vi "CallDLL.vi"() -> ()   [LabVIEW 2013]
uses:
  builds/SenslessProject/Meine DLL/SharedLib.dll
  Windows/System32/kernel32.dll
panel:
  out "String":string
  out "Fehler (Ausgang) 2":errorcluster caption="Fehler (Ausgang)"
  out "arg2":u32
  out "arg1":u32
  out "Fehler (Ausgang)":errorcluster
  out "Rückgabetyp":i32
  out "string_ 2":string
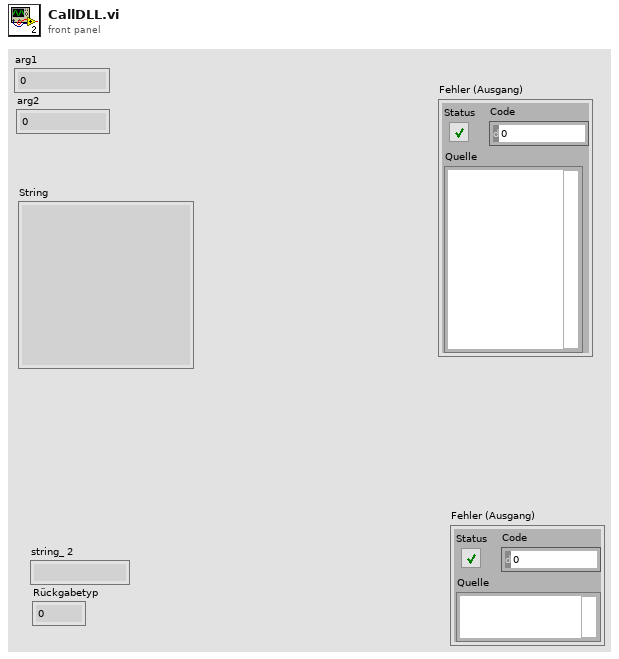
[diagram p1: front panel]
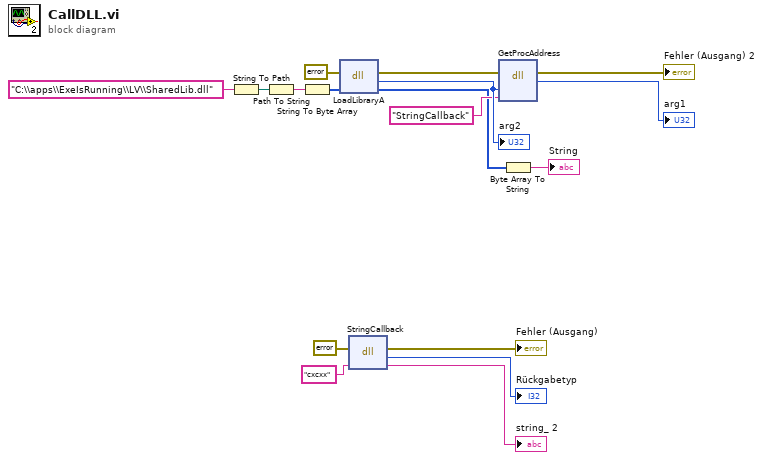
[diagram p0: block diagram]
diagram:
  n1 = String To Path(string="C:\\apps\\ExeIsRunning\\LV\\SharedLib.dll" ("arg1")) -> (path=w14:path)
  n2 = Path To String(path=w14) -> (string=w16:string)
  n3 = String To Byte Array(string=w16) -> (unsigned byte array=w17:u8[])
  n4 = dll-call lib="C:/Windows/System32/kernel32.dll" fn="LoadLibraryA"(error in=errorcluster {"status"=FALSE, "code"=0, "source"=""} ("Fehler (Eingang, kein Fehler)"), "arg1"=w17) -> (error out=w10:errorcluster, "Rückgabetyp"=w13:u32, "arg1"=w3:u8[])  [unwired: 2 in, 1 out]
  "arg2" <- w13
  n5 = dll-call lib="C:/apps/ExeIsRunning/builds/SenslessProject/Meine DLL/SharedLib.dll" fn="StringCallback"(error in=errorcluster {"status"=FALSE, "code"=0, "source"=""} ("Fehler (Eingang, kein Fehler)"), "string_"="cxcxx") -> (error out=→"Fehler (Ausgang)":errorcluster, "Rückgabetyp"=→"Rückgabetyp":i32, "string_"=→"string_ 2":string)  [unwired: 2 in, 1 out]
  n6 = dll-call lib="C:/Windows/System32/kernel32.dll" fn="GetProcAddress"(error in=w10, "arg1"=w13, "arg2"="StringCallback") -> (error out=→"Fehler (Ausgang) 2":errorcluster, "Rückgabetyp"=→"arg1":u32)  [unwired: 4 in, 1 out]
  n7 = Byte Array To String(unsigned byte array=w3) -> (string=→"String":string)
